vi "BASE DETECTION.vi"() -> ()   [LabVIEW 2015]
uses:
  <vilib>/userdefined/High Color/IMAQdx.ctl
  <vilib>/vision/driver/NI_Vision_Acquisition_Software.lvlib
  <resource>/objmgr/imaqdx.rc
  <vilib>/vision/NI_Vision_Development_Module.lvlib
panel:
  out "Image":T1(plugin-control)
  in  "Color Mode":u16(ring) items=["RGB", "HSL", "HSV", "HSI"]
  in  "stop":bool
  out "Image Pixels (Float)":sgl[][](array[numeric]) format="%.2f"
  out "Y Resoloution  2":i32
  out "X Resoloution 2":i32
  out "Video Modes":string
  in  "Video Mode":dbl min=0.0 max=5.0 step=1.0
  in  "Camera":T2
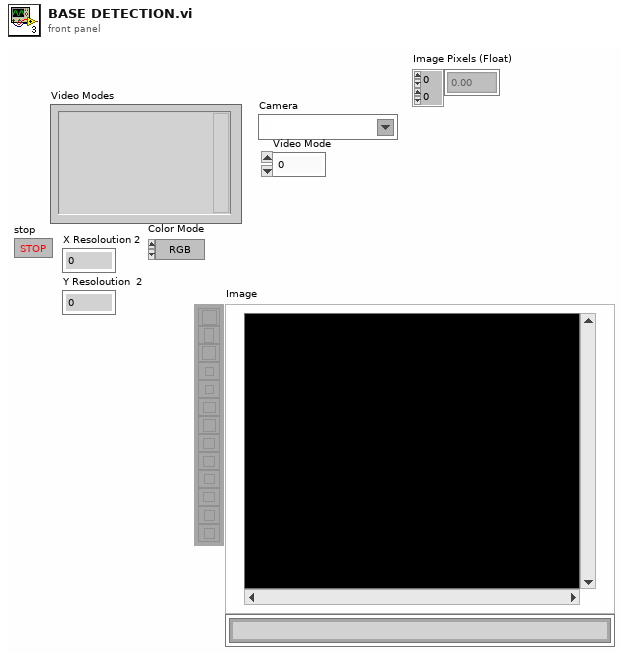
[diagram p1: front panel]
types:
  T1 = typedef "IMAQ Image.ctl" = refnum<image>
  T2 = typedef "IMAQdx.ctl" = refnum<k21>
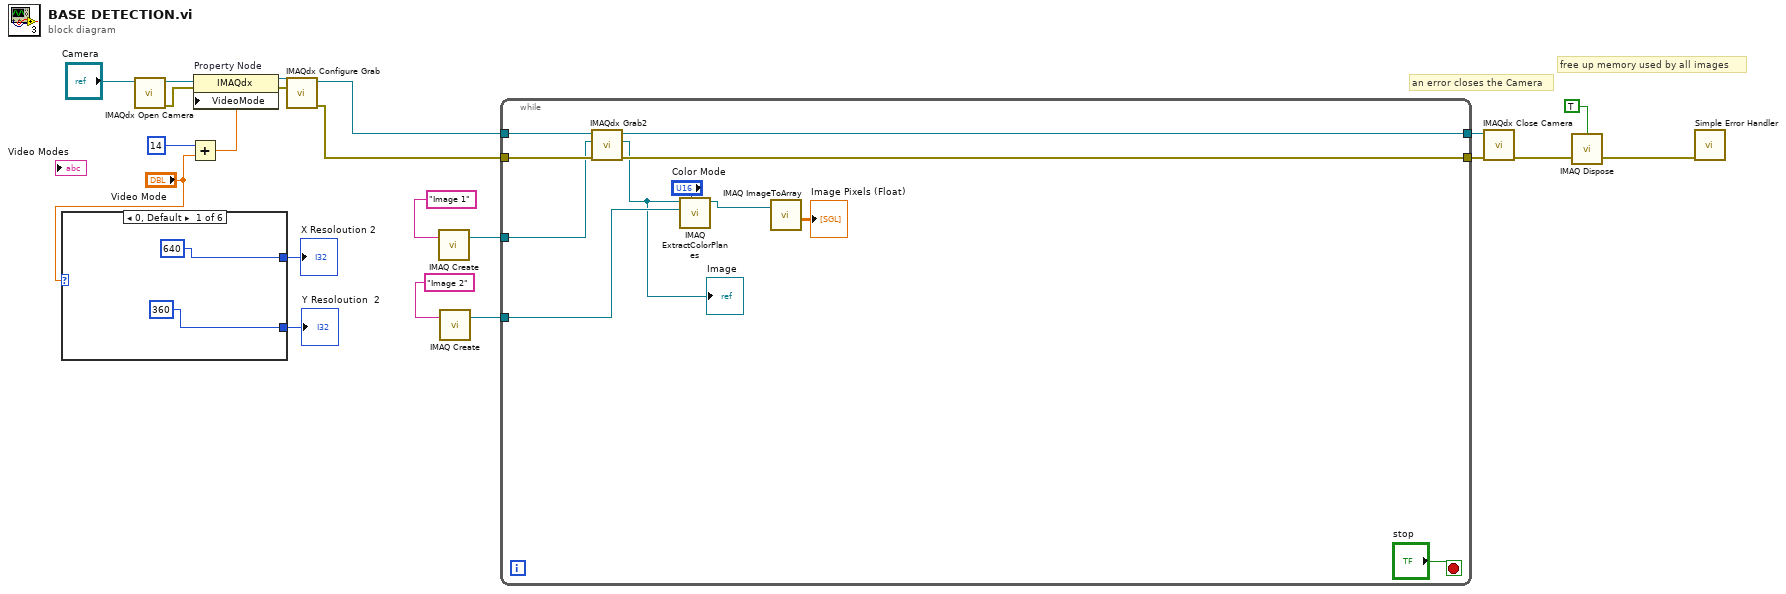
[diagram p0: block diagram]
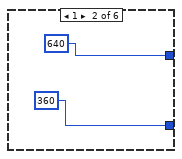
[diagram p2: hidden frame]
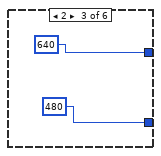
[diagram p3: hidden frame]
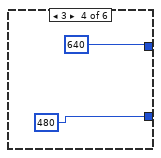
[diagram p4: hidden frame]
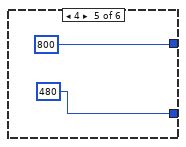
[diagram p5: hidden frame]
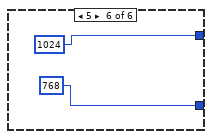
[diagram p6: hidden frame]
diagram:
  # "an error closes the Camera"
  # "free up memory used by all images"
  n1 = case shown="0, Default" "Video Mode" {
    tunnel: [640 640 640 640 800 1024] -> w11
    tunnel: [360 360 480 480 480 768] -> w10
    frame 0, Default {
    }
    frame 1 {
    }
    frame 2 {
    }
    frame 3 {
    }
    frame 4 {
    }
    frame 5 {
    }
  }
  "X Resoloution 2" <- w11
  "Y Resoloution  2" <- w10
  n2 = call <vilib>:"IMAQdx Open Camera.vi"("Session In"="Camera") -> ("error out"=w18:errorcluster, "Session Out"=w19:T2)  [unwired: 9 in]
  n3 = Add(x=14, y="Video Mode") -> (x+y=w13:dbl)
  n4 = property on="Property Node" class="IMAQdx"(reference=w19, error in=w18, "VideoMode"=w13) -> (reference out=w17:T2, error out=w16:errorcluster)
  n5 = call <vilib>:"IMAQdx Configure Grab.vi"("error in"=w16, "Session In"=w17) -> ("error out"=w8:errorcluster, "Session Out"=w9:T2)  [unwired: 8 in]
  n6 = call "IMAQ Create"("Image Name"="Image 1") -> ("New Image"=w7:T1)  [unwired: 4 in, 1 out]
  n7 = call "IMAQ Create"("Image Name"="Image 2") -> ("New Image"=w1:T1)  [unwired: 4 in, 1 out]
  n8 = while {
    tunnel: w9 -> [w44]
    tunnel: w8 -> [w43]
    tunnel: w7 -> [w42]
    tunnel: [w41] -> w3
    tunnel: [w40] -> w2
    tunnel: w1 -> [w35]
    stop <- "stop" stop-if-true
    n9 = call <vilib>:"IMAQdx Grab2.vi"("error in"=w43, "Image In"=w42, "Session In"=w44) -> ("error out"=w40:errorcluster, "Image Out"=w34:T1, "Session Out"=w41:T2)  [unwired: 5 in, 1 out]
    "Image" <- w34
    n10 = call "IMAQ ExtractColorPlanes"("Color Mode"="Color Mode", "Red or Hue Plane"=w35, "Image Src"=w34) -> ("Red or Hue Plane out"=w39:T1)  [unwired: 5 in, 3 out]
    n11 = call "IMAQ ImageToArray"("Image"=w39) -> ("Image Pixels (Float)"=→"Image Pixels (Float)":sgl[][])  [unwired: 3 in, 4 out]
  }
  n12 = call <vilib>:"IMAQdx Close Camera.vi"("error in"=w2, "Session In"=w3) -> ("error out"=w4:errorcluster)  [unwired: 9 in]
  n13 = call "IMAQ Dispose"("All Images? (No)"=TRUE, "error in (no error)"=w4) -> ("error out"=w5:errorcluster)  [unwired: 4 in]
  n14 = call <vilib>:"Simple Error Handler.vi"("error in (no error)"=w5) -> ()  [unwired: 4 in, 5 out]
